vi "String - Extract Unique Headers_.vi"(11 "Array In":string[](array[string])) -> (3 "Array Out":string[](array[string]))   [LabVIEW 2013]
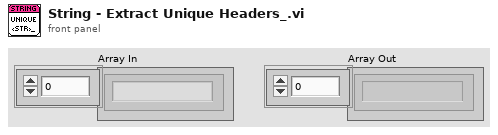
[diagram p1: front panel]
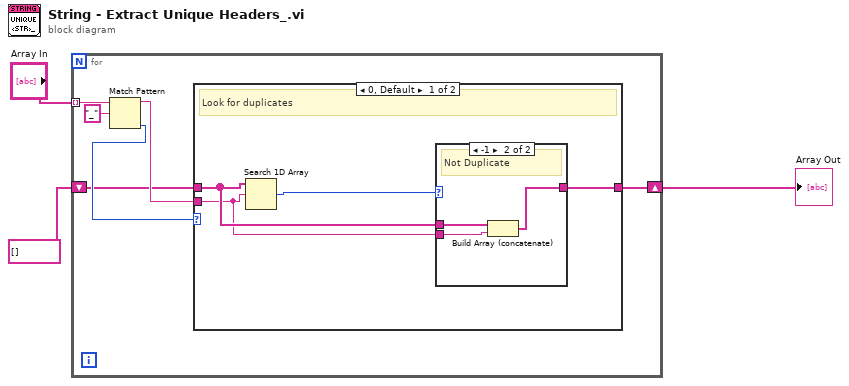
[diagram p0: block diagram]
diagram:
  n1 = for {
    tunnel: "Array In" -> [w9] mode=indexing
    shift-right: [w7] -> w3
    shift-left: string[] [] -> [w4]
    n2 = Match Pattern(string=w9, regular expression="_") -> (before substring=w5:string, offset past match=w6:i32)  [unwired: 1 in, 2 out]
    n3 = case shown="0, Default" w6 {
      tunnel: [w10 w18] -> w7
      tunnel: w5 -> [w11 _]
      tunnel: w4 -> [w12 w18]
      frame 0, Default {
        # "Look for duplicates"
        n4 = Search 1D Array(1D array=w12, element=w11) -> (index of element=w13:i32)  [unwired: 1 in]
        n5 = case shown="-1" w13 {
          tunnel: w12 -> [w14 w17]
          tunnel: w11 -> [_ w16]
          tunnel: [w14 w15] -> w10
          frame 0, Default {
            # "Duplicate"
          }
          frame -1 {
            # "Not Duplicate"
            n6 = Build Array (concatenate)(w17, w16) -> (w15:string[])
          }
        }
      }
      frame -1 {
        # "Not Found"
      }
    }
  }
  "Array Out" <- w3
